vi "Number to binary format.vi"(7 "length in bytes (3)":i32=3, 11 "Numeric":u32) -> (3 "Binary format":string)   [LabVIEW 2019]
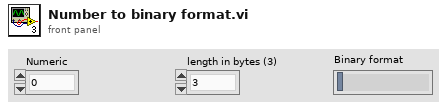
[diagram p1: front panel]
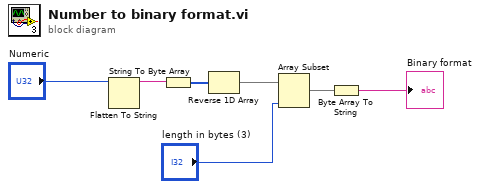
[diagram p0: block diagram]
diagram:
  n1 = Flatten To String(anything="Numeric") -> (data string=w7:string)  [unwired: 3 in, 2 out]
  n2 = String To Byte Array(string=w7) -> (unsigned byte array=w6:u8[])
  n3 = Reverse 1D Array(array=w6) -> (reversed array=w5:u8[])
  n4 = Array Subset(array=w5, length="length in bytes (3)") -> (w4:u8[])  [unwired: 1 in]
  n5 = Byte Array To String(unsigned byte array=w4) -> (string=→"Binary format":string)
